vi "BMU诊断标定.vi"(5 "timeout":u32, 6 "Socket":dbl, 7 "通用配置?":bool, 8 "CAN端口":u16(ring), 9 "设备索引号":u16(ring), 10 "CAN卡类型":u32(ring)=21, 11 "从板号":u8=1) -> (3 "成功?":bool)   [LabVIEW 2013] (continued)
                    n3177 = case shown="\"从板\"" w4302 {
                      tunnel: [0.0 ("FUNC") w4312] -> w4303
                      frame "主板", Default {
                      }
                      frame "从板" {
                        n3178 = local read "从板号"() -> (w4312:u8)
                      }
                    }
                    n3179 = local read "设备索引号"() -> (w4305:u16)
                    n3180 = local read "CAN卡类型"() -> (w4306:u32)
                    n3181 = local read "CAN端口"() -> (w4304:u16)
                    n3182 = call "标定授权发送.vi"("CAN卡类型"=w4306, "解锁类型"=enum16{"读取", "写", "下载"}."写", "设备索引号"=w4305, "CAN端口"=w4304, "是否连接"=TRUE, "板选择"=0, "FUNC"=w4303) -> ("发送成功"=w4310:bool)  [unwired: 8 out]
                  }
                }
                n3183 = case shown="真" w4296 {
                  tunnel: w4300 -> [w4314 w4318]
                  tunnel: w4299 -> [w4313 w4317]
                  tunnel: [w4314 w4320] -> w4298
                  tunnel: [w4313 w4319] -> w4297
                  frame False {
                  }
                  frame True {
                    n3184 = Flush Queue(queue=w4318, error in (no error)=w4317) -> (queue out=w4316:refnum<queue>, error out=w4315:errorcluster)  [unwired: 1 out]
                    n3185 = Enqueue Element(queue=w4316, element="全部写入" ("元素"), error in (no error)=w4315) -> (queue out=w4320:refnum<queue>, error out=w4319:errorcluster)  [unwired: 1 in, 1 out]
                  }
                }
                n3186 = global write "EV05全局变量1.vi" "读取超时"(w4294) -> ()
                n3187 = global write "EV05全局变量1.vi" "流控帧"(w4294) -> ()
                n3188 = local write "消除"(w4293) -> ()
                n3189 = local write "控制1"(w4293) -> ()
                n3190 = global write "EV05全局变量1.vi" "流控帧 2"(w4293) -> ()
                n3191 = local write "写?"(w4293) -> ()
              }
            }
          }
          event "单个读取": Value Change {
            n3192 = event-data() -> ("NewVal"=w4326:bool)  [unwired: 5 out]
            n3193 = case shown="真" w4326 {
              tunnel: w4325 -> [w4328 w4336]
              tunnel: w4324 -> [w4327 w4335]
              tunnel: [w4328 w4334] -> w4323
              tunnel: [w4327 w4333] -> w4322
              frame False {
              }
              frame True {
                w4329 = FALSE ("流控帧")
                w4330 = TRUE ("流控帧 2")
                n3194 = global read "EV05全局变量1.vi" "授权功能"() -> (w4331:bool)
                n3195 = case shown="假" w4331 {
                  tunnel: [TRUE ("发送成功") w4345] -> w4332
                  frame False {
                  }
                  frame True {
                    n3196 = local read "设备索引号"() -> (w4339:u16)
                    n3197 = local read "CAN卡类型"() -> (w4340:u32)
                    n3198 = local read "CAN端口"() -> (w4338:u16)
                    n3199 = call "标定授权发送.vi"("CAN卡类型"=w4340, "解锁类型"=enum16{"读取", "写", "下载"}."读取", "设备索引号"=w4339, "CAN端口"=w4338, "是否连接"=TRUE, "板选择"=0, "FUNC"=u32 1) -> ("发送成功"=w4345:bool)  [unwired: 8 out]
                  }
                }
                n3200 = case shown="真" w4332 {
                  tunnel: w4336 -> [w4347 w4351]
                  tunnel: w4335 -> [w4346 w4349]
                  tunnel: [w4347 w4353] -> w4334
                  tunnel: [w4346 w4352] -> w4333
                  frame False {
                  }
                  frame True {
                    n3201 = Flush Queue(queue=w4351, error in (no error)=w4349) -> (queue out=w4350:refnum<queue>, error out=w4348:errorcluster)  [unwired: 1 out]
                    n3202 = Enqueue Element(queue=w4350, element="单个读取" ("元素"), error in (no error)=w4348) -> (queue out=w4353:refnum<queue>, error out=w4352:errorcluster)  [unwired: 2 out]
                  }
                }
                n3203 = global write "EV05全局变量1.vi" "写入超时"(w4329) -> ()
                n3204 = global write "EV05全局变量1.vi" "流控帧"(w4329) -> ()
                n3205 = local write "写?"(w4329) -> ()
                n3206 = local write "消除"(w4330) -> ()
                n3207 = local write "控制1"(w4330) -> ()
                n3208 = global write "EV05全局变量1.vi" "流控帧 2"(w4330) -> ()
              }
            }
          }
          event "全部读取": Value Change {
            n3209 = event-data() -> ("NewVal"=w4359:bool)  [unwired: 5 out]
            n3210 = case shown="真" w4359 {
              tunnel: w4358 -> [w4361 w4365]
              tunnel: w4357 -> [w4360 w4364]
              tunnel: [w4361 w4363] -> w4356
              tunnel: [w4360 w4362] -> w4355
              frame False {
              }
              frame True {
                n3211 = stacked-sequence {
                  seq-local: [w4370 _] -> [_ _]
                  seq-local: [w4369 _] -> [_ _]
                  tunnel: w4365 -> [w4372 w4402]
                  tunnel: w4364 -> [w4371 w4401]
                  tunnel: [_ w4406] -> w4363
                  tunnel: [_ w4405] -> w4362
                  frame #0 {
                    w4366 = FALSE ("布尔")
                    n3212 = local read "路径"() -> (w4368:path)
                    n3213 = Empty String/Path?(string/path=w4368) -> (empty?=w4367:bool)
                    n3214 = case shown="假" w4367 {
                      tunnel: w4372 -> [w4380 w4398]
                      tunnel: w4371 -> [w4379 w4397]
                      tunnel: [w4376 w4397] -> w4370
                      tunnel: [w4375 w4398] -> w4369
                      frame False {
                        n3215 = global read "EV05全局变量1.vi" "授权功能"() -> (w4377:bool)
                        n3216 = case shown="真" w4377 {
                          tunnel: [TRUE ("发送成功") w4389] -> w4378
                          frame False {
                          }
                          frame True {
                            n3217 = local read "设备索引号"() -> (w4383:u16)
                            n3218 = local read "CAN卡类型"() -> (w4384:u32)
                            n3219 = local read "CAN端口"() -> (w4382:u16)
                            n3220 = call "标定授权发送.vi"("CAN卡类型"=w4384, "解锁类型"=enum16{"读取", "写", "下载"}."读取", "设备索引号"=w4383, "CAN端口"=w4382, "是否连接"=TRUE, "板选择"=0, "FUNC"=u32 1) -> ("发送成功"=w4389:bool)  [unwired: 8 out]
                          }
                        }
                        n3221 = case shown="真" w4378 {
                          tunnel: w4380 -> [w4391 w4396]
                          tunnel: w4379 -> [w4390 w4395]
                          tunnel: [w4391 w4393] -> w4375
                          tunnel: [w4390 w4392] -> w4376
                          frame False {
                          }
                          frame True {
                            n3222 = Enqueue Element(queue=w4396, element="读配置文件" ("元素"), error in (no error)=w4395) -> (queue out=w4393:refnum<queue>, error out=w4392:errorcluster)  [unwired: 2 out]
                          }
                        }
                        n3223 = local write "布尔"(FALSE ("布尔")) -> ()
                        n3224 = Wait Until Next ms Multiple(millisecond multiple=u32 200 ("毫秒倍数")) -> ()  [unwired: 1 out]
                      }
                      frame True {
                      }
                    }
                    n3225 = local write "1 6"(w4366) -> ()
                    n3226 = local write "1 7"(w4366) -> ()
                    n3227 = local write "1 8"(w4366) -> ()
                    n3228 = local write "1 9"(w4366) -> ()
                    n3229 = local write "1 10"(w4366) -> ()
                    n3230 = local write "1 12"(w4366) -> ()
                  }
                  frame #1 {
                    w4399 = FALSE ("流控帧")
                    w4400 = TRUE ("流控帧 2")
                    n3231 = global read "EV05全局变量1.vi" "授权功能"() -> (w4403:bool)
                    n3232 = case shown="假" w4403 {
                      tunnel: [TRUE ("发送成功") w4415] -> w4404
                      frame False {
                      }
                      frame True {
                        n3233 = local read "设备索引号"() -> (w4409:u16)
                        n3234 = local read "CAN卡类型"() -> (w4410:u32)
                        n3235 = local read "CAN端口"() -> (w4408:u16)
                        n3236 = call "标定授权发送.vi"("CAN卡类型"=w4410, "解锁类型"=enum16{"读取", "写", "下载"}."读取", "设备索引号"=w4409, "CAN端口"=w4408, "是否连接"=TRUE, "板选择"=0, "FUNC"=u32 1) -> ("发送成功"=w4415:bool)  [unwired: 8 out]
                      }
                    }
                    n3237 = case shown="真" w4404 {
                      tunnel: w4402 -> [w4417 w4418]
                      tunnel: w4401 -> [w4416 w4421]
                      tunnel: [w4417 w4423] -> w4406
                      tunnel: [w4416 w4422] -> w4405
                      frame False {
                      }
                      frame True {
                        n3238 = Flush Queue(queue=w4418, error in (no error)=w4421) -> (queue out=w4419:refnum<queue>, error out=w4420:errorcluster)  [unwired: 1 out]
                        n3239 = Enqueue Element(queue=w4419, element="全部读取" ("元素"), error in (no error)=w4420) -> (queue out=w4423:refnum<queue>, error out=w4422:errorcluster)  [unwired: 2 out]
                      }
                    }
                    n3240 = global write "EV05全局变量1.vi" "写入超时"(w4399) -> ()
                    n3241 = global write "EV05全局变量1.vi" "流控帧"(w4399) -> ()
                    n3242 = local write "写?"(w4399) -> ()
                    n3243 = local write "消除"(w4400) -> ()
                    n3244 = local write "控制1"(w4400) -> ()
                    n3245 = global write "EV05全局变量1.vi" "流控帧 2"(w4400) -> ()
                  }
                }
              }
            }
          }
          event "开启均衡": Value Change {
            n3246 = event-data() -> ("NewVal"=w4429:bool)  [unwired: 5 out]
            n3247 = case shown="真" w4429 {
              tunnel: w4428 -> [w4431 w4438]
              tunnel: w4427 -> [w4430 w4437]
              tunnel: [w4431 w4436] -> w4426
              tunnel: [w4430 w4435] -> w4425
              frame False {
              }
              frame True {
                n3248 = global read "EV05全局变量1.vi" "授权功能"() -> (w4433:bool)
                n3249 = case shown="假" w4433 {
                  tunnel: [TRUE ("发送成功") w4448] -> w4434
                  frame False {
                  }
                  frame True {
                    n3250 = local read "主从选择"() -> (w4440:enum32{"主板", "从板"})
                    n3251 = case shown="\"从板\"" w4440 {
                      tunnel: [0.0 ("FUNC") w4450] -> w4441
                      frame "主板", Default {
                      }
                      frame "从板" {
                        n3252 = local read "从板号"() -> (w4450:u8)
                      }
                    }
                    n3253 = local read "设备索引号"() -> (w4443:u16)
                    n3254 = local read "CAN卡类型"() -> (w4444:u32)
                    n3255 = local read "CAN端口"() -> (w4442:u16)
                    n3256 = call "标定授权发送.vi"("CAN卡类型"=w4444, "解锁类型"=enum16{"读取", "写", "下载"}."写", "设备索引号"=w4443, "CAN端口"=w4442, "是否连接"=TRUE, "板选择"=0, "FUNC"=w4441) -> ("发送成功"=w4448:bool)  [unwired: 8 out]
                  }
                }
                n3257 = case shown="真" w4434 {
                  tunnel: w4438 -> [w4452 w4457]
                  tunnel: w4437 -> [w4451 w4456]
                  tunnel: [w4452 w4454] -> w4436
                  tunnel: [w4451 w4453] -> w4435
                  frame False {
                  }
                  frame True {
                    n3258 = Enqueue Element(queue=w4457, element="开启均衡" ("元素"), error in (no error)=w4456) -> (queue out=w4454:refnum<queue>, error out=w4453:errorcluster)  [unwired: 2 out]
                  }
                }
                n3259 = call <vilib>:"Set Busy.vi"("disable click? (T)"=TRUE) -> ()  [unwired: 3 in, 8 out]
              }
            }
          }
          event "关闭均衡": Value Change {
            n3260 = event-data() -> ("NewVal"=w4462:bool)  [unwired: 5 out]
            n3261 = case shown="真" w4462 {
              tunnel: w4461 -> [w4464 w4471]
              tunnel: w4460 -> [w4463 w4470]
              tunnel: [w4464 w4469] -> w4459
              tunnel: [w4463 w4468] -> w4458
              frame False {
              }
              frame True {
                n3262 = global read "EV05全局变量1.vi" "授权功能"() -> (w4466:bool)
                n3263 = case shown="假" w4466 {
                  tunnel: [TRUE ("发送成功") w4481] -> w4467
                  frame False {
                  }
                  frame True {
                    n3264 = local read "主从选择"() -> (w4473:enum32{"主板", "从板"})
                    n3265 = case shown="\"从板\"" w4473 {
                      tunnel: [0.0 ("FUNC") w4483] -> w4474
                      frame "主板", Default {
                      }
                      frame "从板" {
                        n3266 = local read "从板号"() -> (w4483:u8)
                      }
                    }
                    n3267 = local read "设备索引号"() -> (w4476:u16)
                    n3268 = local read "CAN卡类型"() -> (w4477:u32)
                    n3269 = local read "CAN端口"() -> (w4475:u16)
                    n3270 = call "标定授权发送.vi"("CAN卡类型"=w4477, "解锁类型"=enum16{"读取", "写", "下载"}."写", "设备索引号"=w4476, "CAN端口"=w4475, "是否连接"=TRUE, "板选择"=0, "FUNC"=w4474) -> ("发送成功"=w4481:bool)  [unwired: 8 out]
                  }
                }
                n3271 = case shown="真" w4467 {
                  tunnel: w4471 -> [w4485 w4490]
                  tunnel: w4470 -> [w4484 w4489]
                  tunnel: [w4485 w4487] -> w4469
                  tunnel: [w4484 w4486] -> w4468
                  frame False {
                  }
                  frame True {
                    n3272 = Enqueue Element(queue=w4490, element="关闭均衡" ("元素"), error in (no error)=w4489) -> (queue out=w4487:refnum<queue>, error out=w4486:errorcluster)  [unwired: 2 out]
                  }
                }
                n3273 = call <vilib>:"Set Busy.vi"("disable click? (T)"=TRUE) -> ()  [unwired: 3 in, 8 out]
              }
            }
          }
          event "强制开启均衡": Value Change {
            n3274 = event-data() -> ("NewVal"=w4495:bool)  [unwired: 5 out]
            n3275 = case shown="真" w4495 {
              tunnel: w4494 -> [w4497 w4504]
              tunnel: w4493 -> [w4496 w4503]
              tunnel: [w4497 w4502] -> w4492
              tunnel: [w4496 w4501] -> w4491
              frame False {
              }
              frame True {
                n3276 = global read "EV05全局变量1.vi" "授权功能"() -> (w4499:bool)
                n3277 = case shown="假" w4499 {
                  tunnel: [TRUE ("发送成功") w4514] -> w4500
                  frame False {
                  }
                  frame True {
                    n3278 = local read "主从选择"() -> (w4506:enum32{"主板", "从板"})
                    n3279 = case shown="\"从板\"" w4506 {
                      tunnel: [0.0 ("FUNC") w4516] -> w4507
                      frame "主板", Default {
                      }
                      frame "从板" {
                        n3280 = local read "从板号"() -> (w4516:u8)
                      }
                    }
                    n3281 = local read "设备索引号"() -> (w4509:u16)
                    n3282 = local read "CAN卡类型"() -> (w4510:u32)
                    n3283 = local read "CAN端口"() -> (w4508:u16)
                    n3284 = call "标定授权发送.vi"("CAN卡类型"=w4510, "解锁类型"=enum16{"读取", "写", "下载"}."写", "设备索引号"=w4509, "CAN端口"=w4508, "是否连接"=TRUE, "板选择"=0, "FUNC"=w4507) -> ("发送成功"=w4514:bool)  [unwired: 8 out]
                  }
                }
                n3285 = case shown="真" w4500 {
                  tunnel: w4504 -> [w4518 w4523]
                  tunnel: w4503 -> [w4517 w4522]
                  tunnel: [w4518 w4520] -> w4502
                  tunnel: [w4517 w4519] -> w4501
                  frame False {
                  }
                  frame True {
                    n3286 = Enqueue Element(queue=w4523, element="强制均衡" ("元素"), error in (no error)=w4522) -> (queue out=w4520:refnum<queue>, error out=w4519:errorcluster)  [unwired: 2 out]
                  }
                }
                n3287 = call <vilib>:"Set Busy.vi"("disable click? (T)"=TRUE) -> ()  [unwired: 3 in, 8 out]
              }
            }
          }
        }
        n3288 = local read "停止"() -> (w1728:bool)
        n3289 = Or(x=w1727, y=w1728) -> (x .or. y?=w1726:bool)
      }
      n3290 = Release Queue(queue=w1723, force destroy? (F)=TRUE ("强制销毁？(F)"), error in (no error)=w1722) -> (error out=w1720:errorcluster)  [unwired: 2 out]
      n3291 = call <vilib>:"Clear Errors.vi"("error in (no error)"=w1720) -> ()  [unwired: 7 out]
    }
    frame Disabled {
    }
  }
  n3292 = case shown="无错误" w49 {
    tunnel: w14 -> [w4526 _]
    tunnel: w13 -> [w4525 _]
    tunnel: w1 -> [w4524 _]
    frame No Error {
      n3293 = case shown="\"全部写入\"" "全部写入" {
        tunnel: w4526 -> [_ _ w4659 _ _ _ _ _ _ _ _ _ _ _ _]
        tunnel: w4525 -> [_ _ w4658 _ _ _ _ _ _ _ _ _ _ _ _]
        tunnel: w4524 -> [_ _ w4657 _ _ _ _ _ _ _ _ _ _ _ _]
        frame "假", Default {
          n3294 = local write "强制终止读写标记"(FALSE ("强制终止读写标记")) -> ()
        }
        frame "单个写入" {
          n3295 = local read "主从选择"() -> (w4535:enum32{"主板", "从板"})
          n3296 = case shown="\"从板\"" w4535 {
            tunnel: [w4546 w4561] -> w4532
            tunnel: [0.0 w4559] -> w4536
            tunnel: [_ w4560] -> w4534
            tunnel: [w4544 _] -> w4533
            frame "主板", Default {
              n3297 = stacked-sequence {
                tunnel: [_ w4558] -> w4544
                frame #0 {
                  n3298 = control-ref of="高压参数"() -> (w4549:refnum<vi>)
                  n3299 = control-ref of="电池信息"() -> (w4550:refnum<vi>)
                  n3300 = control-ref of="一级故障"() -> (w4556:refnum<vi>)
                  n3301 = control-ref of="一级故障 2"() -> (w4554:refnum<vi>)
                  n3302 = control-ref of="一级故障 3"() -> (w4553:refnum<vi>)
                  n3303 = control-ref of="加热控制参数"() -> (w4552:refnum<vi>)
                  n3304 = control-ref of="充电控制参数"() -> (w4551:refnum<vi>)
                  n3305 = control-ref of="项目信息"() -> (w4555:refnum<vi>)
                  n3306 = control-ref of="项目信息2"() -> (w4557:refnum<vi>)
                  n3307 = local read "主板数据"() -> (w4547:T4)
                  n3308 = Bundle(cluster=w4547, "项目信息"=w4555, "一级故障 4"=w4557, "一级故障"=w4556, "一级故障 2"=w4554, "一级故障 3"=w4553, "加热控制参数"=w4552, "充电控制参数"=w4551, "高压参数"=w4549, "电池信息"=w4550) -> (w4548:T4)
                  n3309 = local write "主板数据"(w4548) -> ()
                }
                frame #1 {
                  n3310 = control-ref of="主板数据"() -> (w4558:refnum<vi>)
                }
              }
              n3311 = local read "主板选项"() -> (w4546:string)
            }
            frame "从板" {
              n3312 = stacked-sequence {
                tunnel: [_ w4572] -> w4560
                frame #0 {
                  n3313 = control-ref of="从板号"() -> (w4571:refnum<vi>)
                  n3314 = control-ref of="项目信息 2"() -> (w4570:refnum<vi>)
                  n3315 = control-ref of="均衡参数"() -> (w4565:refnum<vi>)
                  n3316 = control-ref of="加热控制参数"() -> (w4569:refnum<vi>)
                  n3317 = control-ref of="一级故障(从板)"() -> (w4568:refnum<vi>)
                  n3318 = control-ref of="二级故障(从板)"() -> (w4567:refnum<vi>)
                  n3319 = control-ref of="三级故障(从板)"() -> (w4566:refnum<vi>)
                  n3320 = control-ref of="电池组信息"() -> (w4562:refnum<vi>)
                  n3321 = local read "从板信息"() -> (w4563:T2)
                  n3322 = Bundle(cluster=w4563, "从板号"=w4571, "项目信息 2"=w4570, "加热控制参数"=w4569, "一级故障(从板)"=w4568, "二级故障(从板)"=w4567, "三级故障(从板)"=w4566, "电池组信息(从板)"=w4562, "均衡参数"=w4565) -> (w4564:T2)
                  n3323 = local write "从板信息"(w4564) -> ()
                }
                frame #1 {
                  n3324 = control-ref of="从板信息"() -> (w4572:refnum<vi>)
                }
              }
              n3325 = local read "从板选项"() -> (w4561:string)
              n3326 = local read "从板号"() -> (w4559:u8)
            }
          }
          n3327 = local read "从板个数"() -> (w4537:dbl)
          n3328 = local read "快换"() -> (w4538:bool)
          n3329 = call "输入数据解析.vi"("单个参数补充"=w4537, "从板号"=w4536, "主板引用"=w4533, "从板引用"=w4534, "主板选项"=w4532, "枚举"=w4535, "快换"=w4538) -> ("输出数组"=w4542:dbl[][], "数组长度"=w4541:dbl[], "循环次数"=w4531:i32, "命令"=w4540:u32, "名称"=w4530:string[], "命令序号"=w4539:u32[])  [unwired: 2 in, 1 out]
          n3330 = for {
            N: w4531 -> [w4578]
            tunnel: w4542 -> [w4588]
            tunnel: w4541 -> [w4587]
            tunnel: w4540 -> [w4586]
            tunnel: w4539 -> [w4585]
            tunnel: w4536 -> [w4576]
            tunnel: w4532 -> [w4584]
            tunnel: w4530 -> [w4580]
            tunnel: [w4573] -> w4529
            i -> [w4579]
            n3331 = Index Array(array=w4588, index (row)=w4579) -> (element=w4583:dbl[])  [unwired: 1 in]
            n3332 = Index Array(array=w4587, index=w4579) -> (element=w4582:dbl)
            n3333 = Index Array(array=w4580, index=w4579) -> (element=w4577:string)
            n3334 = case shown="\"从板号\"" w4577 {
              tunnel: [w4590 w4591] -> w4575
              tunnel: w4576 -> [w4590 _]
              tunnel: [TRUE ("确定") w4592] -> w4574
              frame "假", Default {
              }
              frame "从板号" {
                n3335 = call "请输入当前从板板号"() -> ("当前从板板号"=w4591:dbl, "确定"=w4592:bool)  [unwired: 17 in, 1 out]
                n3336 = local write "当前从板板号"(w4591) -> ()
              }
            }
            n3337 = Index Array(array=w4585, index=w4579) -> (element=w4581:u32)
            n3338 = global write "全局 1.vi" "名称"(w4577) -> ()
            n3339 = case shown="真" w4574 {
              tunnel: w4586 -> [_ w4602]
              tunnel: w4584 -> [_ w4601]
              tunnel: w4583 -> [_ w4600]
              tunnel: w4582 -> [_ w4599]
              tunnel: w4581 -> [_ w4598]
              tunnel: w4579 -> [_ w4597]
              tunnel: w4577 -> [_ w4596]
              tunnel: w4578 -> [_ w4595]
              tunnel: w4575 -> [_ w4594]
              tunnel: [_ w4593] -> w4573
              frame False {
                n3340 = call <vilib>:"Unset Busy.vi"() -> ()  [unwired: 11 in, 1 out]
              }
              frame True {
                n3341 = stacked-sequence {
                  seq-local: [_ _ _ w4630 _ _] -> [_ _ _ _ w4639 _]
                  tunnel: w4600 -> [_ _ w4615 _ _ _]
                  tunnel: w4599 -> [_ _ w4614 _ _ _]
                  tunnel: w4602 -> [_ _ w4608 _ _ _]
                  tunnel: w4598 -> [_ _ w4606 _ _ _]
                  tunnel: w4601 -> [_ _ _ _ _ _]
                  tunnel: w4597 -> [_ _ _ _ _ w4650]
                  tunnel: w4596 -> [_ _ _ _ w4638 _]
                  tunnel: w4595 -> [_ _ _ _ _ w4651]
                  tunnel: w4594 -> [_ _ w4607 _ _ _]
                  tunnel: [_ _ _ _ _ w4648] -> w4593
                  frame #0 {
                    w4604 = FALSE ("流控帧")
                    w4603 = TRUE ("流控帧 2")
                    n3342 = global write "EV05全局变量1.vi" "读取超时"(w4604) -> ()
                    n3343 = global write "EV05全局变量1.vi" "流控帧"(w4604) -> ()
                    n3344 = local write "消除"(w4603) -> ()
                    n3345 = local write "控制1"(w4603) -> ()
                    n3346 = global write "EV05全局变量1.vi" "流控帧 2"(w4603) -> ()
                    n3347 = local write "写?"(w4603) -> ()
                  }
                  frame #1 {
                    n3348 = Wait Until Next ms Multiple(millisecond multiple=u32 50 ("毫秒倍数")) -> ()  [unwired: 1 out]
                  }
                  frame #2 {
                    n3349 = local read "设备索引号"() -> (w4610:u16)
                    n3350 = local read "CAN卡类型"() -> (w4611:u32)
                    n3351 = Increment(x=w4614) -> (x+1=w4613:dbl)
                    n3352 = local read "CAN端口"() -> (w4609:u16)
                    n3353 = local write "命令"(w4608) -> ()
                    n3354 = local write "命令序号"(w4606) -> ()
                    n3355 = Reshape Array(w4615, w4613) -> (w4612:dbl[])
                    n3356 = stacked-sequence {
                      tunnel: w4612 -> [_ w4629]
                      tunnel: w4611 -> [w4618 w4628]
                      tunnel: w4610 -> [w4617 w4627]
                      tunnel: w4609 -> [w4616 w4626]
                      tunnel: w4608 -> [_ w4625]
                      tunnel: w4607 -> [_ w4624]
                      tunnel: w4606 -> [_ w4623]
                      frame #0 {
                        n3357 = disable-structure shown="禁用" {
                          disable-tunnel: w4618 -> [w4621 _]
                          disable-tunnel: w4617 -> [w4620 _]
                          disable-tunnel: w4616 -> [w4619 _]
                          frame Disabled {
                            n3358 = dll-call lib="PTH1abs FBluewave New EnergySVN_WorkAutoTest_TestStandtrunkAutoTest_TestStandDriverZlgCanBHN01è¯»ååæ°data\nkerneldlls\nusbcan.dll" fn="VCI_ClearBuffer"("DeviceType"=w4621, "DeviceInd"=w4620, "CANInd"=w4619) -> (error out=w4622:errorcluster)  [unwired: 4 in, 4 out]
                            n3359 = call <vilib>:"Clear Errors.vi"("error in (no error)"=w4622) -> ()  [unwired: 6 in, 1 out]
                          }
                          frame Enabled {
                          }
                        }
                      }
                      frame #1 {
                        n3360 = call "多帧发送机制(EV05).vi"("can卡类型"=w4628, "设备索引号"=w4627, "CAN端口"=w4626, "命令"=w4625, "板号"=w4624, "命令序号"=w4623, "输入数据"=w4629) -> ()  [unwired: 2 in, 11 out]
                      }
                    }
                  }
                  frame #3 {
                    n3361 = while {
                      tunnel: [w4632] -> w4630
                      i -> [w4636]
                      stop <- w4633 stop-if-true
                      n3362 = local read "强制终止读写标记"() -> (w4631:bool)
                      n3363 = global read "EV05全局变量1.vi" "读取超时"() -> (w4632:bool)
                      n3364 = Greater Or Equal?(x=w4636, y=30) -> (x >= y?=w4634:bool)
                      n3365 = Wait Until Next ms Multiple(millisecond multiple=u32 100 ("毫秒倍数")) -> ()  [unwired: 1 out]
                      n3366 = Compound Arithmetic op=OR(w4631, w4632, w4634) -> (w4633:bool)
                    }
                  }
                  frame #4 {
                    n3367 = case shown="假" w4639 {
                      tunnel: w4638 -> [w4640 w4646]
                      frame False {
                        n3368 = control-ref of="结果"() -> (w4644:refnum<vi>)
                        n3369 = Concatenate Strings(w4640, "       写入失败" ("字符串")) -> (w4643:string)
                        n3370 = Build Array(w4643) -> (w4642:string[])
                        n3371 = call "表格编辑.vi"("新元素/子数组"=w4642, "活动单元格:单元格背景色"=u32 16740749, "MCListbox引用句柄"=w4644) -> ()  [unwired: 9 out]
                      }
                      frame True {
                        n3372 = case shown="\"从板号\"" w4646 {
                          frame "假", Default {
                          }
                          frame "从板号" {
                            n3373 = local read "从板号"() -> (w4647:u8)
                            n3374 = local write "当前从板板号"(w4647) -> ()
                          }
                        }
                      }
                    }
                  }
                  frame #5 {
                    n3375 = Increment(x=w4650) -> (x+1=w4649:i32)
                    n3376 = Equal?(x=w4651, y=w4649) -> (x = y?=w4648:bool)
                    n3377 = case shown="真" w4648 {
                      frame False {
                      }
                      frame True {
                        n3378 = control-ref of="结果"() -> (w4655:refnum<vi>)
                        n3379 = Concatenate Strings("写入完成" ("字符串")) -> (w4654:string)
                        n3380 = Build Array(w4654) -> (w4653:string[])
                        n3381 = call "表格编辑.vi"("新元素/子数组"=w4653, "活动单元格:单元格背景色"=u32 21937, "MCListbox引用句柄"=w4655) -> ()  [unwired: 9 out]
                      }
                    }
                  }
                }
              }
            }
          }
          n3382 = stacked-sequence {
            tunnel: w4529 -> [_]
            frame #0 {
              n3383 = call <vilib>:"Unset Busy.vi"() -> ()  [unwired: 2 in, 10 out]
              n3384 = local write "强制终止读写标记"(FALSE ("强制停止")) -> ()
            }
          }
        }
        frame "全部写入" {
          n3385 = local read "主从选择"() -> (w4665:enum32{"主板", "从板"})
          n3386 = case shown="\"从板\"" w4665 {
            tunnel: [string[] ["项目信息", "一级故障阀值", "二级故障阀值", "三级故障阀值", "加热控制参数", "充电控制参数", "电池信息", "二维码"] w4892] -> w4662
            tunnel: [0.0 ("从板号") w4890] -> w4666
            tunnel: [w4873 _] -> w4664
            tunnel: [_ w4891] -> w4663
            tunnel: w4659 -> [_ w4890]
            frame "主板", Default {
              n3387 = stacked-sequence {
                tunnel: [_ w4887] -> w4873
                frame #0 {
                  n3388 = control-ref of="电池信息"() -> (w4879:refnum<vi>)
                  n3389 = control-ref of="高压参数"() -> (w4878:refnum<vi>)
                  n3390 = control-ref of="一级故障"() -> (w4881:refnum<vi>)
                  n3391 = control-ref of="一级故障 2"() -> (w4883:refnum<vi>)
                  n3392 = control-ref of="一级故障 3"() -> (w4884:refnum<vi>)
                  n3393 = control-ref of="加热控制参数"() -> (w4885:refnum<vi>)
                  n3394 = control-ref of="充电控制参数"() -> (w4886:refnum<vi>)
                  n3395 = control-ref of="项目信息"() -> (w4882:refnum<vi>)
                  n3396 = control-ref of="项目信息2"() -> (w4880:refnum<vi>)
                  n3397 = local read "主板数据"() -> (w4877:T4)
                  n3398 = Bundle(cluster=w4877, "项目信息"=w4882, "一级故障 4"=w4880, "一级故障"=w4881, "一级故障 2"=w4883, "一级故障 3"=w4884, "加热控制参数"=w4885, "充电控制参数"=w4886, "高压参数"=w4878, "电池信息"=w4879) -> (w4876:T4)
                  n3399 = local write "主板数据"(w4876) -> ()
                }
                frame #1 {
                  n3400 = control-ref of="主板数据"() -> (w4887:refnum<vi>)
                }
              }
            }
            frame "从板" {
              (unwired) "均衡参数"
              n3401 = local read "通用配置?"() -> (w4888:bool)
              n3402 = case shown="假" w4888 {
                tunnel: [string[] ["从板信息", "一级故障阀值", "二级故障阀值", "三级故障阀值"] string[] ["从板信息", "一级故障阀值", "二级故障阀值", "三级故障阀值", "二维码"]] -> w4892
                frame False {
                }
                frame True {
                }
              }
              n3403 = stacked-sequence {
                tunnel: [_ w4905] -> w4891
                frame #0 {
                  n3404 = control-ref of="从板号"() -> (w4899:refnum<vi>)
                  n3405 = control-ref of="项目信息 2"() -> (w4900:refnum<vi>)
                  n3406 = control-ref of="均衡参数"() -> (w4897:refnum<vi>)
                  n3407 = control-ref of="加热控制参数"() -> (w4901:refnum<vi>)
                  n3408 = control-ref of="一级故障(从板)"() -> (w4902:refnum<vi>)
                  n3409 = control-ref of="二级故障(从板)"() -> (w4903:refnum<vi>)
                  n3410 = control-ref of="三级故障(从板)"() -> (w4904:refnum<vi>)
                  n3411 = control-ref of="电池组信息"() -> (w4898:refnum<vi>)
                  n3412 = local read "从板信息"() -> (w4896:T2)
                  n3413 = Bundle(cluster=w4896, "从板号"=w4899, "项目信息 2"=w4900, "加热控制参数"=w4901, "一级故障(从板)"=w4902, "二级故障(从板)"=w4903, "三级故障(从板)"=w4904, "电池组信息(从板)"=w4898, "均衡参数"=w4897) -> (w4895:T2)
                  n3414 = local write "从板信息"(w4895) -> ()
                }
                frame #1 {
                  n3415 = control-ref of="从板信息"() -> (w4905:refnum<vi>)
                }
              }
              n3416 = local write "从板号"(w4890) -> ()
              n3417 = local write "失败？"(FALSE ("失败")) -> ()
            }
          }
          n3418 = Array Size(array=w4662) -> (size(s)=w4661:i32)
          n3419 = for {
            tunnel: w4665 -> [w4678]
            tunnel: w4666 -> [w4681]
            tunnel: w4664 -> [w4680]
            tunnel: w4663 -> [w4679]
            tunnel: w4661 -> [w4673]
            tunnel: [w4672] -> w4660
            tunnel: w4658 -> [w4671]
            tunnel: w4662 -> [w4669] mode=indexing
            tunnel: w4657 -> [w4667]
            i -> [w4674]
            n3420 = local read "二维码"() -> (w4668:string)
            n3421 = disable-structure shown="禁用" {
              disable-tunnel: w4678 -> [w4691 _]
              disable-tunnel: w4674 -> [w4690 _]
              disable-tunnel: w4673 -> [w4689 _]
              disable-tunnel: [w4687 _] -> w4672
              frame Disabled {
                n3422 = Increment(x=w4690) -> (x+1=w4688:i32)
                n3423 = Less Or Equal?(x=w4689, y=w4688) -> (x <= y?=w4687:bool)
                n3424 = case shown="\"从板\"" w4691 {
                  tunnel: w4690 -> [w4693 w4707]
                  frame "主板", Default {
                    n3425 = case shown="6" w4693 {
                      tunnel: [T8."项目信息" ("主从板") T8."一级故障阀值" ("主从板") T8."二级故障阀值" ("主从板") T8."三级故障阀值" ("主从板") T8."控制参数" ("主从板") T8."电池信息" ("主从板")] -> w4692
                      frame 0, Default {
                        n3426 = local write "1"(TRUE ("1")) -> ()
                      }
                      frame 1 {
                        n3427 = local write "1 2"(TRUE ("1 2")) -> ()
                      }
                      frame 2 {
                        n3428 = local write "1 3"(TRUE ("1 3")) -> ()
                      }
                      frame 3 {
                        n3429 = local write "1 4"(TRUE ("1 4")) -> ()
                      }
                      frame 4, 5 {
                        n3430 = local write "1 5"(TRUE ("1 5")) -> ()
                      }
                      frame 6 {
                        n3431 = local write "1 11"(TRUE ("1 11")) -> ()
                      }
                    }
                    n3432 = local write "主板2"(w4692) -> ()
                  }
                  frame "从板" {
                    n3433 = case shown="1" w4707 {
                      tunnel: [T21."从板信息" ("等级 2") T21."从板信息" ("等级 2") T21."一级故障阀值" ("等级 2") T21."二级故障阀值" ("等级 2") T21."三级故障阀值" ("等级 2") T21."快换参数" ("等级 2") T14."均衡参数" ("等级 2")] -> w4706
                      frame 99, Default {
                        n3434 = local write "1 6"(TRUE ("1 6")) -> ()
                      }
                      frame 0 {
                        n3435 = local write "1 6"(TRUE ("1 6")) -> ()
                      }
                      frame 1 {
                        n3436 = local write "1 7"(TRUE ("1 7")) -> ()
                      }
                      frame 2 {
                        n3437 = local write "1 8"(TRUE ("1 8")) -> ()
                      }
                      frame 3 {
                        n3438 = local write "1 9"(TRUE ("1 9")) -> ()
                      }
                      frame 4 {
                        n3439 = local write "1 10"(TRUE ("1 10")) -> ()
                      }
                      frame 5 {
                        n3440 = local write "1 12"(TRUE ("1 10")) -> ()
                      }
                    }
                    n3441 = local write "等级 2"(w4706) -> ()
                  }
                }
              }
              frame Enabled {
              }
            }
            n3442 = local read "从板个数"() -> (w4686:dbl)
            n3443 = local read "快换"() -> (w4677:bool)
            n3444 = call "输入数据解析.vi"("单个参数补充"=w4686, "从板号"=w4681, "从板二维码"=w4668, "主板引用"=w4680, "从板引用"=w4679, "主板选项"=w4669, "枚举"=w4678, "快换"=w4677) -> ("输出数组"=w4685:dbl[][], "数组长度"=w4684:dbl[], "循环次数"=w4676:i32, "命令"=w4683:u32, "名称"=w4675:string[], "命令序号"=w4682:u32[])  [unwired: 1 in, 1 out]
            n3445 = for {
              N: w4676 -> [w4728]
              tunnel: w4685 -> [w4738]
              tunnel: w4684 -> [w4737]
              tunnel: w4683 -> [w4736]
              tunnel: w4682 -> [w4734]
              tunnel: w4681 -> [w4735]
              tunnel: w4675 -> [w4731]
              tunnel: w4672 -> [w4726]
              tunnel: w4669 -> [w4725]
              tunnel: w4671 -> [w4724]
              tunnel: w4667 -> [w4722]
              i -> [w4727]
              n3446 = Index Array(array=w4738, index (row)=w4727) -> (element=w4733:dbl[])  [unwired: 1 in]
              n3447 = Index Array(array=w4737, index=w4727) -> (element=w4732:dbl)
              n3448 = Index Array(array=w4731, index=w4727) -> (element=w4729:string)
              n3449 = Index Array(array=w4734, index=w4727) -> (element=w4730:u32)
              n3450 = local write "重试次数"(u8 0 ("重试次数")) -> ()
              n3451 = while {
                tunnel: w4736 -> [w4753]
                tunnel: w4735 -> [w4752]
                tunnel: w4733 -> [w4751]
                tunnel: w4732 -> [w4750]
                tunnel: w4730 -> [w4749]
                tunnel: w4729 -> [w4748]
                tunnel: w4728 -> [w4747]
                tunnel: w4727 -> [w4746]
                tunnel: w4726 -> [w4745]
                tunnel: w4725 -> [w4744]
                tunnel: w4724 -> [w4743]
                tunnel: w4722 -> [w4739]
                stop <- w4740 stop-if-true
                # "用于重测"
                n3452 = stacked-sequence {
                  seq-local: [_ _ _ w4793 _ _] -> [_ _ _ _ w4819 _]
                  tunnel: w4751 -> [_ _ w4778 _ _ _]
                  tunnel: w4750 -> [_ _ w4777 _ _ _]
                  tunnel: w4753 -> [_ _ w4773 _ _ _]
                  tunnel: w4752 -> [_ _ w4768 _ _ _]
                  tunnel: w4749 -> [_ _ w4774 _ _ _]
                  tunnel: w4748 -> [_ _ w4767 w4792 w4818 _]
                  tunnel: w4747 -> [_ _ _ _ _ w4841]
                  tunnel: w4746 -> [_ _ _ _ _ w4840]
                  tunnel: w4745 -> [_ _ _ _ _ w4838]
                  tunnel: w4744 -> [_ _ _ _ _ _]
                  tunnel: w4743 -> [_ _ w4769 _ _ _]
                  tunnel: [_ _ _ _ w4817 _] -> w4742
                  tunnel: w4739 -> [w4757 _ _ w4791 _ _]
                  frame #0 {
                    w4759 = FALSE ("流控帧")
                    w4758 = TRUE ("流控帧 2")
                    n3453 = global write "EV05全局变量1.vi" "读取超时"(w4759) -> ()
                    n3454 = global write "EV05全局变量1.vi" "流控帧"(w4759) -> ()
                    n3455 = global write "EV05全局变量1.vi" "流控帧 2"(w4758) -> ()
                    n3456 = local write "消除"(w4758) -> ()
                    n3457 = local write "控制1"(w4758) -> ()
                    n3458 = local write "写?"(w4758) -> ()
                    n3459 = call <vilib>:"Acquire Semaphore.vi"("semaphore"=w4757) -> ("error out"=w4756:errorcluster, "semaphore out"=w4755:T24)  [unwired: 4 in, 1 out]
                    n3460 = flat-sequence {
                      tunnel: w4756 -> [_]
                      tunnel: [w4761] -> w4754
                      tunnel: w4755 -> [w4761]
                      frame #0 {
                        n3461 = global read "EV05全局变量1.vi" "写入超时Array"() -> (w4764:bool[])
                        n3462 = local read "Socket"() -> (w4762:dbl)
                        n3463 = local write "读取超时"(FALSE ("读取超时")) -> ()
                        n3464 = Replace Array Subset(array=w4764, new element=FALSE ("写入超时"), index=w4762) -> (w4763:bool[])
                        n3465 = global write "EV05全局变量1.vi" "写入超时Array"(w4763) -> ()
                      }
                    }
                    n3466 = call <vilib>:"Release Semaphore.vi"("semaphore"=w4754) -> ()  [unwired: 5 in, 2 out]
                    "流控帧" <- w4759
                    "流控帧 2" <- w4758
                  }
                  frame #1 {
                    n3467 = Wait Until Next ms Multiple(millisecond multiple=u32 50 ("毫秒倍数")) -> ()  [unwired: 1 out]
                  }
                  frame #2 {
                    n3468 = global write "全局 1.vi" "名称"(w4767) -> ()
                    n3469 = local write "命令"(w4773) -> ()
                    n3470 = Equal?(x=w4767, y="从板号") -> (x = y?=w4770:bool)
                    n3471 = Select(t=w4769, s=w4770, f=w4768) -> (s? t:f=w4772:dbl)
                    n3472 = local write "命令序号"(w4774) -> ()
                    n3473 = local read "CAN卡类型"() -> (w4781:u32)
                    n3474 = local read "设备索引号"() -> (w4780:u16)
                    n3475 = local read "CAN端口"() -> (w4779:u16)
                    n3476 = Increment(x=w4777) -> (x+1=w4775:dbl)
                    n3477 = Reshape Array(w4778, w4775) -> (w4776:dbl[])
                    n3478 = stacked-sequence {
                      tunnel: w4781 -> [_ w4790]
                      tunnel: w4780 -> [_ w4789]
                      tunnel: w4779 -> [_ w4788]
                      tunnel: w4776 -> [_ w4787]
                      tunnel: w4772 -> [_ w4786]
                      tunnel: w4774 -> [_ w4785]
                      tunnel: w4773 -> [_ w4784]
                      frame #0 {
                      }
                      frame #1 {
                        n3479 = control-ref of="流控帧"() -> (w4782:refnum<vi>)
                        n3480 = call "多帧发送机制(EV05).vi"("can卡类型"=w4790, "设备索引号"=w4789, "CAN端口"=w4788, "命令"=w4784, "板号"=w4786, "命令序号"=w4785, "输入数据"=w4787, "流控帧"=w4782) -> ("错误输出"=w4783:errorcluster)  [unwired: 1 in, 10 out]
                        n3481 = call <vilib>:"Clear Errors.vi"("error in (no error)"=w4783) -> ()  [unwired: 6 in, 1 out]
                      }
                    }
                    "Step" <- w4767
                  }
                  frame #3 {
                    n3482 = case shown="\"假\", 默认" w4792 {
                      tunnel: [w4795 TRUE ("读取超时")] -> w4793
                      tunnel: w4791 -> [w4794 _]
                      frame "假", Default {
                        n3483 = while {
                          tunnel: [w4799] -> w4795
                          tunnel: w4794 -> [w4798]
                          i -> [w4805]
                          stop <- w4802 stop-if-true
                          n3484 = local read "强制终止读写标记"() -> (w4800:bool)
                          n3485 = Greater Or Equal?(x=w4805, y=30) -> (x >= y?=w4803:bool)
                          n3486 = Wait Until Next ms Multiple(millisecond multiple=u32 100 ("毫秒倍数")) -> ()  [unwired: 1 out]
                          n3487 = Compound Arithmetic op=OR(w4800, w4799, w4803) -> (w4802:bool)
                          n3488 = call <vilib>:"Acquire Semaphore.vi"("semaphore"=w4798) -> ("semaphore out"=w4797:T24)  [unwired: 4 in, 2 out]
                          n3489 = flat-sequence {
                            tunnel: [w4806] -> w4799
                            tunnel: w4797 -> [w4807]
                            tunnel: [w4807] -> w4796
                            frame #0 {
                              n3490 = local read "读取超时"() -> (w4806:bool)
                              n3491 = global read "EV05全局变量1.vi" "写入超时Array"() -> (w4809:bool[])
                              n3492 = local read "Socket"() -> (w4808:dbl)
                              n3493 = Index Array(array=w4809, index=w4808) -> ()  [unwired: 1 out]
                            }
                          }
                          n3494 = call <vilib>:"Release Semaphore.vi"("semaphore"=w4796) -> ()  [unwired: 5 in, 2 out]
                        }
                      }
                      frame "从板号" {
                        (unwired) u32 9 ("表格总行数")
                        (unwired) 5 ("保留行数")
                        n3495 = global read "全局 1.vi" "名称"() -> (w4815:string)
                        n3496 = control-ref of="结果"() -> (w4810:refnum<vi>)
                        n3497 = Concatenate Strings(w4815, "       写入成功" ("字符串")) -> (w4812:string)
                        n3498 = Build Array(w4812) -> (w4813:string[])
                        n3499 = call "表格编辑.vi"("新元素/子数组"=w4813, "活动单元格:单元格背景色"=u32 6618880, "MCListbox引用句柄"=w4810) -> ()  [unwired: 9 out]
                      }
                    }
                  }
                  frame #4 {
                    n3500 = case shown="假" w4819 {
                      tunnel: w4818 -> [w4821 _]
                      tunnel: [w4820 TRUE] -> w4817
                      frame False {
                        n3501 = local read "重试次数"() -> (w4825:u8)
                        n3502 = Increment(x=w4825) -> (x+1=w4824:u8)
                        n3503 = Greater Or Equal?(x=w4824, y=u8 4) -> (x >= y?=w4822:bool)
                        n3504 = local write "重试次数"(w4824) -> ()
                        n3505 = case shown="真" w4822 {
                          tunnel: w4821 -> [_ w4829]
                          tunnel: [FALSE TRUE] -> w4820
                          frame False {
                          }
                          frame True {
                            n3506 = control-ref of="结果"() -> (w4833:refnum<vi>)
                            n3507 = Concatenate Strings(w4829, "       写入失败" ("字符串")) -> (w4832:string)
                            n3508 = Build Array(w4832) -> (w4831:string[])
                            n3509 = call "表格编辑.vi"("新元素/子数组"=w4831, "活动单元格:单元格背景色"=u32 16740749, "MCListbox引用句柄"=w4833) -> ()  [unwired: 9 out]
                            "失败？" <- TRUE
                          }
                        }
                      }
                      frame True {
                      }
                    }
                  }
                  frame #5 {
                    n3510 = Increment(x=w4840) -> (x+1=w4836:i32)
                    n3511 = Equal?(x=w4841, y=w4836) -> (x = y?=w4839:bool)
                    n3512 = And(x=w4838, y=w4839) -> (x .and. y?=w4837:bool)
                    n3513 = case shown="真" w4837 {
                      frame False {
                      }
                      frame True {
                        n3514 = Concatenate Strings("写入完成" ("字符串")) -> (w4844:string)
                        n3515 = control-ref of="结果"() -> (w4845:refnum<vi>)
                        n3516 = Build Array(w4844) -> (w4843:string[])
                        n3517 = call "表格编辑.vi"("新元素/子数组"=w4843, "活动单元格:单元格背景色"=u32 21937, "MCListbox引用句柄"=w4845) -> ()  [unwired: 9 out]
                      }
                    }
                  }
                }
                n3518 = local read "timeout"() -> (w4741:bool)
                n3519 = Or(x=w4742, y=w4741) -> (x .or. y?=w4740:bool)
              }
            }
            n3520 = local write "重试次数"(u8 0 ("重试次数")) -> ()
          }
          n3521 = stacked-sequence {
            tunnel: [_ w4859 _] -> _
            tunnel: w4660 -> [_ _ _]
            frame #0 {
              n3522 = local read "失败？"() -> (w4848:bool)
              n3523 = Not(x=w4848) -> (.not. x?=→"成功?":bool)
              n3524 = disable-structure shown="禁用" {
                frame Disabled {
                  w4858 = "BMURESULT" ("section")
                  n3525 = call <vilib>:"Open Config Data.vi"("error in (no error)"=errorcluster {"status"=FALSE, "code"=0, "source"=""}, "configuration file path"=path "D:/BlueWay/configresult.ini") -> ("error out"=w4856:errorcluster, "refnum"=w4853:T19)  [unwired: 7 in, 1 out]
                  n3526 = Select(t="FAIL" ("key"), f="PASS" ("key")) -> (s? t:f=w4849:string)  [unwired: 1 in]
                  n3527 = call-poly <vilib>:"Write Key.vi"("section"=w4858, "error in (no error)"=w4856, "value"=w4849, "key"=w4858, "refnum"=w4853) -> ("error out"=w4857:errorcluster, "refnum out"=w4854:T19)  [unwired: 4 in, 1 out]
                  n3528 = call <vilib>:"Close Config Data.vi"("error in (no error)"=w4857, "refnum"=w4854) -> ()  [unwired: 8 in, 2 out]
                }
                frame Enabled {
                }
              }
            }
            frame #1 {
              n3529 = disable-structure shown="禁用" {
                disable-tunnel: [w4860 _] -> w4859
                frame Disabled {
                  w4867 = u8 0 items=["Normal", "Listen Only"] ("工作方式")
                  w4866 = u8 1 items=["Dual Filter", "Single Filter"] ("滤波方式")
                  n3530 = local read "设备索引号"() -> (w4862:u16)
                  n3531 = local read "CAN卡类型"() -> (w4861:u32)
                  n3532 = local read "CAN端口"() -> (w4863:u16)
                  n3533 = call "CAN_Init-8.6.vi"("CAN卡类型"=w4861, "设备索引号"=w4862, "CAN端口"=w4863, "操作类型"=enum16{"初始化CAN", "关闭CAN"}."关闭CAN", "滤波方式"=w4866, "Accept Code"=u32 3221225472, "簇"=T23 {"打开CAN"=FALSE, "初始化CAN"=FALSE, "开始CAN"=FALSE, "重启"=TRUE, "关闭CAN"=TRUE}, "Mask Code"=u32 1073741823 ("Accept Code"), "工作方式"=w4867, "是否滤波"=TRUE, "滤波选择"=T22 {"fiter_mode"=1, "fiter_endid"=402653184, "fiter_startid"=419430399}) -> ("error out"=w4860:errorcluster)  [unwired: 3 in, 5 out]
                }
                frame Enabled {
                }
              }
            }
            frame #2 {
              n3534 = local write "停止"(TRUE ("停止")) -> ()
            }
          }
        }
        frame "单个读取" {
          n3535 = stacked-sequence {
            tunnel: [w4908] -> w4906
            frame #0 {
              n3536 = local read "主从选择"() -> (w4909:enum32{"主板", "从板"})
              n3537 = case shown="\"主板\", 默认" w4909 {
                tunnel: [w4922 w5002] -> w4911
                tunnel: [w4921 w5003] -> w4916
                tunnel: [0 ("从板号") w4999] -> w4915
                tunnel: [0 ("板号") u8 0 ("板号")] -> w4914
                tunnel: [w4917 w4998] -> w4912
                frame "主板", Default {
                  n3538 = local read "主板选项"() -> (w4918:string)
                  n3539 = case shown="\"SOC过低(3)\", \"SOC过高(3)\", \"SOH过低(3)\", \"充电电流过高(3)\", \"单体电压过低(3)\", \"单体电压过高(3)\", \"单组电压不均衡(3)\", \"单组温度不均衡(3)\", \"放电电流过高(3)\", \"极柱温度过高(3)\", \"内阻过大(3)\", \"三级故障阀值\", \"温度过低(3)\", \"温度过高(3)\", \"整组电压不均衡(3)\", \"整组温度不均衡(3)\", \"总电压过低(3)\", \"总电压过高(3)\"" w4918 {
                    tunnel: [_ u8[] [1, 2, 3, 4, 5, 6, 13, 8, 7, 9, 10, 11, 12] u8[] [1] u8[] [1] u8[] [2] u8[] [3] u8[] [4] u8[] [5] u8[] [6] u8[] [13] u8[] [7] u8[] [8] u8[] [9] u8[] [10] u8[] [14] u8[] [11] u8[] [12] u8[] [2] u8[] [3] u8[] [1] u8[] [2] u8[] [1] u8[] [2] u8[] [3] u8[] [4] u8[] [1, 2, 3, 4]] -> w4922
                    tunnel: [_ u8 128 ("命令") u8 129 ("命令") u8 128 ("命令") u8 128 ("命令") u8 128 ("命令") u8 128 ("命令") u8 128 ("命令") u8 128 ("命令") u8 128 ("命令") u8 128 ("命令") u8 128 ("命令") u8 128 ("命令") u8 128 ("命令") u8 128 ("命令") u8 128 ("命令") u8 128 ("命令") u8 129 ("命令") u8 129 ("命令") u8 130 ("命令") u8 130 ("命令") u8 132 ("命令") u8 132 ("命令") u8 132 ("命令") u8 132 ("命令") u8 132 ("命令")] -> w4921
                    tunnel: [_ string[] ["产品编号", "电压个数", "通道电压数", "电压起始值", "温度个数", "温度起始值", "保险位置", "电池额定实际容量", "SOC", "配置文件版本", "参数修改记录", "车牌号", "SOH"] string[] ["一级故障阀值"] string[] ["产品编号"] string[] ["电压个数"] string[] ["通道电压数"] string[] ["电压起始值"] string[] ["温度个数"] string[] ["温度起始值"] string[] ["保险位置"] string[] ["SOC"] string[] ["电池额定实际容量"] string[] ["配置文件版本"] string[] ["参数修改记录"] string[] ["校正时钟"] string[] ["车牌号"] string[] ["SOH"] string[] ["二级故障阀值"] string[] ["三级故障阀值"] string[] ["加热控制参数"] string[] ["充电控制参数"] string[] ["电池信息1"] string[] ["电池包组号"] string[] ["充放电安时"] string[] ["电池充放电次数"] string[] ["电池信息1", "电池包组号", "充放电安时", "电池充放电次数"]] -> w4917
                    frame "假", Default {
                    }
                    frame "项目信息" {
                    }
                    frame "SOC过低", "SOC过高", "SOH过低", "充电电流过高", "单体电压过低", "单体电压过高", "单组电压不均衡", "单组温度不均衡", "放电电流过高", "极柱温度过高", "内阻过大", "温度过低", "温度过高", "一级故障阀值", "整组电压不均衡", "整组温度不均衡", "总电压过低", "总电压过高" {
                    }
                    frame "产品编号" {
                    }
                    frame "电压个数" {
                    }
                    frame "通道电压数" {
                    }
                    frame "电压起始值" {
                    }
                    frame "温度个数" {
                    }
                    frame "温度起始值" {
                    }
                    frame "保险位置" {
                    }
                    frame "SOC" {
                    }
                    frame "电池额定实际容量" {
                    }
                    frame "配置文件版本" {
                    }
                    frame "参数修改记录" {
                    }
                    frame "校正时钟" {
                    }
                    frame "车牌号" {
                    }
                    frame "SOH" {
                    }
                    frame "SOC过低(2)", "SOC过高(2)", "SOH过低(2)", "充电电流过高(2)", "单体电压过低(2)", "单体电压过高(2)", "单组电压不均衡(2)", "单组温度不均衡(2)", "二级故障阀值", "放电电流过高(2)", "极柱温度过高(2)", "内阻过大(2)", "温度过低(2)", "温度过高(2)", "整组电压不均衡(2)", "整组温度不均衡(2)", "总电压过低(2)", "总电压过高(2)" {
                    }
                    frame "SOC过低(3)", "SOC过高(3)", "SOH过低(3)", "充电电流过高(3)", "单体电压过低(3)", "单体电压过高(3)", "单组电压不均衡(3)", "单组温度不均衡(3)", "放电电流过高(3)", "极柱温度过高(3)", "内阻过大(3)", "三级故障阀值", "温度过低(3)", "温度过高(3)", "整组电压不均衡(3)", "整组温度不均衡(3)", "总电压过低(3)", "总电压过高(3)" {
                    }
                    frame "风机关闭温差", "风机关闭温度", "风机开启温差", "风机开启温度", "加热关闭温差", "加热关闭温度", "加热开启温度", "加热控制参数" {
                    }
                    frame "充电控制参数", "电流步长", "最大允许充电电流", "最大允许充电温度", "最大允许单体电压", "最大允许总电压", "最小允许充电电流", "最小允许充电温度", "最小允许单体电压" {
                    }
                    frame "电池信息1" {
                    }
                    frame "电池包组号" {
                    }
                    frame "充放电安时" {
                    }
                    frame "电池充放电次数" {
                    }
                    frame "电池信息" {
                    }
                  }
                }
                frame "从板" {
                  n3540 = local read "从板选项"() -> (w5000:string)
                  n3541 = case shown="\"从板信息\"" w5000 {
                    tunnel: [_ u8 0 ("命令") u8 0 ("命令") u8 0 ("命令") u8 0 ("命令") u8 0 ("命令") u8 0 ("命令") u8 0 ("命令") u8 2 ("命令") u8 2 ("命令") u8 2 ("命令") u8 3 ("命令") u8 6 ("命令") u8 6 ("命令") u8 6 ("命令") u8 3 ("命令") u8 3 ("命令") u8 3 ("命令") u8 3 ("命令") u8 3 ("命令") u8 3 ("命令") u8 3 ("命令")] -> w5003
                    tunnel: [_ u8[] [6] u8[] [6, 1, 2, 3, 4, 5] u8[] [1] u8[] [2] u8[] [3] u8[] [4] u8[] [5] u8[] [1] u8[] [2] u8[] [3] u8[] [1, 2, 3, 4, 5, 6, 7] u8[] [1, 2] u8[] [2] u8[] [1] u8[] [1] u8[] [2] u8[] [3] u8[] [4] u8[] [5] u8[] [6] u8[] [7]] -> w5002
                    tunnel: [_ string[] ["从板号"] string[] ["从板号", "电压起始值", "通道电压个数", "保险位置", "温度起始值", "加热控制参数"] string[] ["电压起始值"] string[] ["通道电压节数"] string[] ["保险位置"] string[] ["温度起始值"] string[] ["加热控制参数"] string[] ["一级故障阀值"] string[] ["二级故障阀值"] string[] ["三级故障阀值"] string[] ["电池包信息1", "电池包序号", "充放电安时", "充电次数时间", "SOC", "车牌号", "充电参数"] string[] ["均衡阀值", "充电结束电压"] string[] ["充电结束电压"] string[] ["均衡阀值"] string[] ["电池包信息1"] string[] ["电池包序号"] string[] ["充放电安时"] string[] ["充电次数时间"] string[] ["SOC"] string[] ["车牌号"] string[] ["充电参数"]] -> w4998
                    frame "假", Default {
                    }
                    frame "从板号" {
                    }
